vi "Robo Team Update Controller Setup INI.vi"(11 "Controller Setup":T1={"Pitch Ratio"=1, "Roll Ratio"=1, "Yaw Ratio"=1, "Host IP"="", "Yaw Exist?"=FALSE, "Acceleration"=60000, "Hold Current"=5, "Run Current"=50, "Velocity"=10000, "Pitch Gain"=3000, "Roll Gain"=-3000, "Homing at Startup?"=FALSE, "Extended Logging"=FALSE, "VelocityY"=10000} {"Yaw Ratio" min=1; "Roll Ratio" min=1; "Pitch Ratio" min=1}) -> (0 "error out":errorcluster)   [LabVIEW 2015]
uses:
  Robo Team Controller Setup.ctl
  LP Globals.vi
  <vilib>/Utility/config.llb/Write Key (I32).vi
  <vilib>/Utility/config.llb/Write Key (String).vi
  <vilib>/Utility/config.llb/Write Key (Boolean).vi
  <vilib>/Utility/config.llb/NI_LVConfig.lvlib
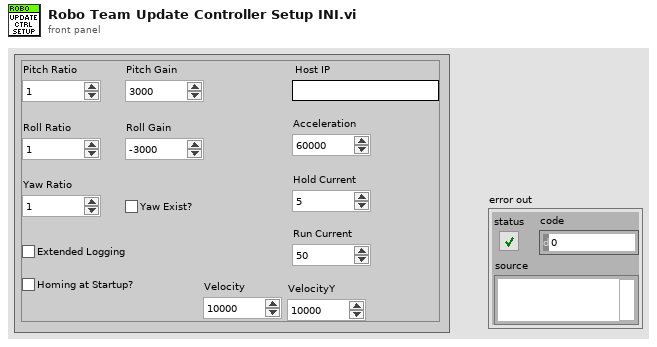
[diagram p1: front panel]
types:
  T1 = typedef "Robo Team Controller Setup.ctl" = cluster{"Pitch Ratio":i32, "Roll Ratio":i32, "Yaw Ratio":i32, "Host IP":string, "Yaw Exist?":bool, "Acceleration":i32, "Hold Current":i32, "Run Current":i32, "Velocity":i32, "Pitch Gain":i32, "Roll Gain":i32, "Homing at Startup?":bool, "Extended Logging":bool, "VelocityY":i32}
  T2 = typedef "NI_LVConfig.lvlib/Config Data RefNum.ctl" = refnum<k1>
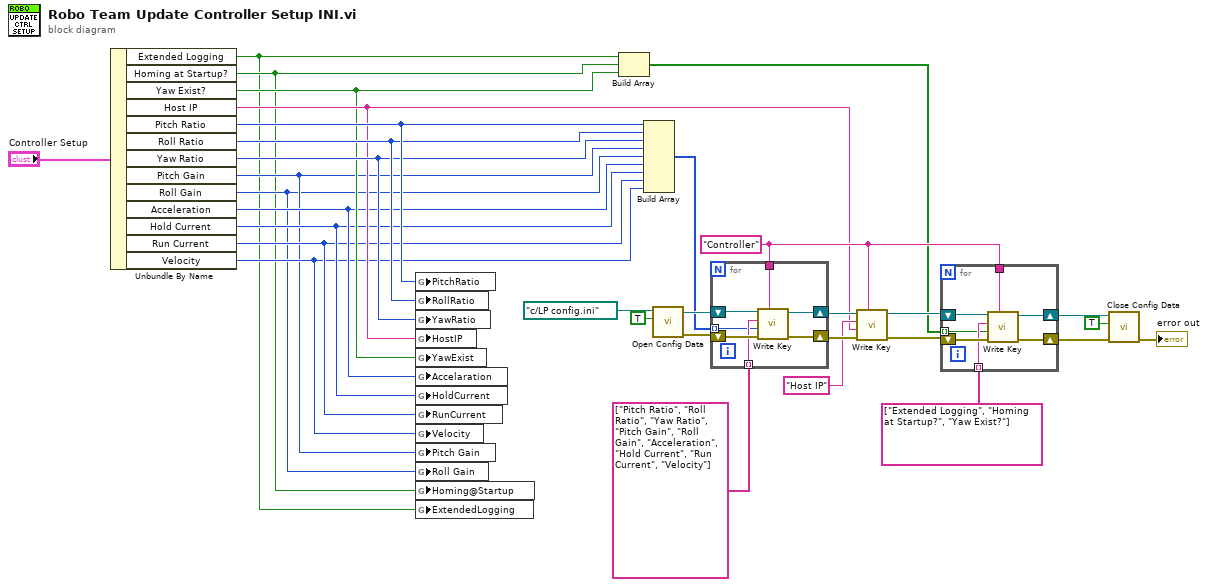
[diagram p0: block diagram]
diagram:
  w20 = "Controller" ("section")
  n1 = Unbundle By Name("Controller Setup") -> ("Extended Logging"=w1:bool, "Homing at Startup?"=w2:bool, "Yaw Exist?"=w9:bool, "Host IP"=w10:string, "Pitch Ratio"=w13:i32, "Roll Ratio"=w12:i32, "Yaw Ratio"=w11:i32, "Pitch Gain"=w4:i32, "Roll Gain"=w3:i32, "Acceleration"=w8:i32, "Hold Current"=w7:i32, "Run Current"=w6:i32, "Velocity"=w5:i32)
  n2 = global write "LP Globals.vi" "PitchRatio"(w13) -> ()
  n3 = global write "LP Globals.vi" "RollRatio"(w12) -> ()
  n4 = global write "LP Globals.vi" "YawRatio"(w11) -> ()
  n5 = global write "LP Globals.vi" "HostIP"(w10) -> ()
  n6 = global write "LP Globals.vi" "YawExist"(w9) -> ()
  n7 = global write "LP Globals.vi" "Accelaration"(w8) -> ()
  n8 = global write "LP Globals.vi" "HoldCurrent"(w7) -> ()
  n9 = global write "LP Globals.vi" "RunCurrent"(w6) -> ()
  n10 = global write "LP Globals.vi" "Velocity"(w5) -> ()
  n11 = global write "LP Globals.vi" "Pitch Gain"(w4) -> ()
  n12 = global write "LP Globals.vi" "Roll Gain"(w3) -> ()
  n13 = global write "LP Globals.vi" "Homing@Startup"(w2) -> ()
  n14 = global write "LP Globals.vi" "ExtendedLogging"(w1) -> ()
  n15 = Build Array(w1, w2, w9) -> (w15:bool[])
  n16 = Build Array(w13, w12, w11, w4, w3, w8, w7, w6, w5) -> (w16:i32[])
  n17 = call <vilib>:"Open Config Data.vi"("create file if necessary (T)"=TRUE, "configuration file path"=path "c:/LP config.ini") -> ("error out"=w18:errorcluster, "refnum"=w19:T2)  [unwired: 7 in, 1 out]
  n18 = for {
    tunnel: string[] ["Pitch Ratio", "Roll Ratio", "Yaw Ratio", "Pitch Gain", "Roll Gain", "Acceleration", "Hold Current", "Run Current", "Velocity"] -> [w37] mode=indexing
    shift-right: [w36] -> w27
    shift-left: w19 -> [w38]
    shift-right: [w35] -> w28
    shift-left: w18 -> [w39]
    tunnel: w20 -> [w34]
    tunnel: w16 -> [w33] mode=indexing
    n19 = call-poly <vilib>:"Write Key.vi"("section"=w34, "error in (no error)"=w39, "value"=w33, "key"=w37, "refnum"=w38) -> ("error out"=w35:errorcluster, "refnum out"=w36:T2)  [unwired: 4 in, 1 out]
  }
  n20 = call-poly <vilib>:"Write Key.vi"("section"=w20, "error in (no error)"=w28, "value"=w10, "key"="Host IP", "refnum"=w27) -> ("error out"=w22:errorcluster, "refnum out"=w23:T2)  [unwired: 4 in, 1 out]
  n21 = for {
    tunnel: string[] ["Extended Logging", "Homing at Startup?", "Yaw Exist?"] -> [w44] mode=indexing
    shift-right: [w43] -> w25
    shift-left: w23 -> [w45]
    shift-right: [w42] -> w24
    shift-left: w22 -> [w46]
    tunnel: w20 -> [w41]
    tunnel: w15 -> [w40] mode=indexing
    n22 = call-poly <vilib>:"Write Key.vi"("section"=w41, "error in (no error)"=w46, "value"=w40, "key"=w44, "refnum"=w45) -> ("error out"=w42:errorcluster, "refnum out"=w43:T2)  [unwired: 4 in, 1 out]
  }
  n23 = call <vilib>:"Close Config Data.vi"("error in (no error)"=w24, "write file if changed (T)"=TRUE, "refnum"=w25) -> ("error out"=→"error out":errorcluster)  [unwired: 7 in, 1 out]
